vi "参数设置页.vi"() -> ()   [LabVIEW 2016, in "斯坦道总氮.lvlib"]
uses:
  <vilib>/Plasmionique/MB Master/MB_Master/MB_Master.lvclass
panel:
  in  "通讯连接":bool
  out "MB table":enum32{"Serial", "TCP"}(tab)
  in  "请选择串口:":refnum<visa-resource-name>
  in  "IP":string="127.0.0.1"
  in  "PORT":string="1001"
  in  "通信方式选择":enum16{"串口", "TCP"}(ring)
  in  "盐度自动补偿：":bool
  out "盐度补偿值":dbl caption="盐度补偿值："
  in  "刷新":bool
  in  "测量模式":enum16{"水样测量", "零点核查", "跨度核查", "标样核查", "加标回收"}(ring)
  in  "参数下拉列表":u16(ring)
  in  "量程下拉列表":enum16{"低量程", "高量程"}(ring)
  in  "流程路径":path=path "data/流程.xml"
  in  "标样核查量程模式":enum16{"高量程", "低量程", "自动"}(ring) caption="标样核查量程模式："
  in  "加标回收量程模式":enum16{"高量程", "低量程", "自动"}(ring) caption="加标回收量程模式："
  in  "跨度核查量程模式":enum16{"高量程", "低量程", "自动"}(ring) caption="跨度核查量程模式："
  in  "零点核查量程模式":enum16{"高量程", "低量程", "自动"}(ring) caption="零点核查量程模式："
  in  "水样测试量程模式":enum16{"高量程", "低量程", "自动"}(ring) caption="水样测试量程模式："
  out "稀释度":dbl caption="稀释度："
  out "阈值（高->低）":dbl caption="阈值（高->低）："
  out "阈值（低->高）":dbl caption="阈值（低->高）："
  out "量程下限":dbl caption="量程下限："
  out "量程上限":dbl caption="量程上限："
  out "检出限":dbl caption="检出限："
  out "曲线截距":dbl caption="曲线截距：" format="%#.6f"
  out "曲线斜率":dbl caption="曲线斜率：" format="%#.6f"
  out "二次多项式系数":dbl caption="二次多项式系数：" format="%#.6f"
  out "消解时长":dbl caption="消解时长："
  out "消解温度":dbl caption="消解温度："
  out "测量精度":u16 caption="测量精度："
  in  "标样核查标液浓度":dbl caption="标样核查标液浓度："
  in  "跨度核查标液浓度":dbl caption="跨度核查标液浓度："
  in  "零点核查标液浓度":dbl caption="零点核查标液浓度："
  in  "跨度值":dbl caption="跨度值："
  # "ppt"
  # "mg/L"
  # "mg/L"
  # "mg/L"
  # "mg/L"
  # "mg/L"
  # "min"
  # "℃"
  # "mg/L"
  # "mg/L"
  # "mg/L"
  # "mg/L"
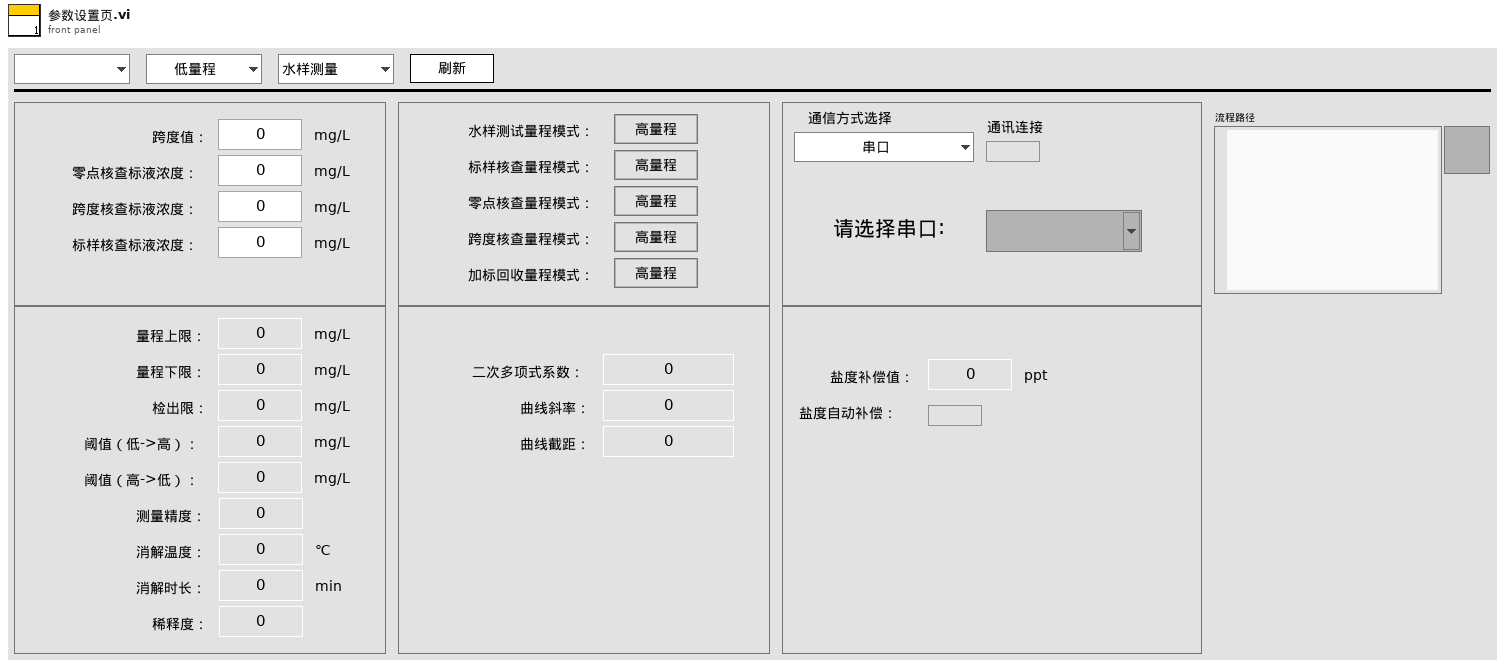
[diagram p1: front panel]
types:
  T1 = typedef "LVStringsAndValuesArrayTypeDef_U16.ctl" = cluster{"String":string, "Value":u16}[]
  T2 = enum8{"Enabled", "Disabled", "Disabled and Grayed Out"}
  T3 = cluster{"泵类型":u8, "进样速度":u32, "出样速度":u32, "泵阀量":u8, "光谱仪类型":u8, "光谱采样次数":u8, "氙灯次数":u8, "B":u16, "C":u16, "D":u16, "E":u16, "B_COD":u16, "C_COD":u16, "D_COD":u16, "E_COD":u16, "G":u16, "M":u16, "N":u16, "氨氮注射泵控温下限":sgl, "氨氮注射泵控温上限":sgl, "总氮注射泵控温下限":sgl, "总氮注射泵控温上限":sgl, "消解温度下限":sgl, "消解温度上限":sgl, "加热10s限值":sgl, "高温高压阀开阀温度":sgl, "总氮x公式0":u8, "总氮x公式1":sgl, "总氮x公式2":sgl, "总磷浊度稀释系数":sgl, "总磷浊度补偿权重1":sgl, "总磷浊度补偿权重2":sgl, "盐度系数":sgl, "氨氮补偿系数1":sgl, "氨氮补偿系数2":sgl}
  T4 = cluster{"测量精度":u16, "检出限":dbl, "上限":dbl, "下限":dbl, "阈值（低->高）":dbl, "阈值（高->低）":dbl, "稀释度":dbl}
  T5 = cluster{"水样测试量程模式":enum16{"高量程", "低量程", "自动"}, "零点核查量程模式":enum16{"高量程", "低量程", "自动"}, "跨度核查量程模式":enum16{"高量程", "低量程", "自动"}, "加标回收量程模式":enum16{"高量程", "低量程", "自动"}, "标样核查量程模式":enum16{"高量程", "低量程", "自动"}}
  T6 = cluster{"总磷跨度值":dbl, "总磷零点标准液浓度":dbl, "总磷跨度标准液浓度":dbl, "总磷标准液标准浓度":dbl, "总氮跨度值":dbl, "总氮零点标准液浓度":dbl, "总氮跨度标准液浓度":dbl, "总氮标准液标准浓度":dbl, "COD跨度值":dbl, "COD零点标准液浓度":dbl, "COD跨度标准液浓度":dbl, "COD标准液标准浓度":dbl, "氨氮跨度值":dbl, "氨氮零点标准液浓度":dbl, "氨氮跨度标准液浓度":dbl, "氨氮标准液标准浓度":dbl, "磷酸盐跨度值":dbl, "磷酸盐零点标准液浓度":dbl, "磷酸盐跨度标准液浓度":dbl, "磷酸盐标准液标准浓度":dbl, "硝氮跨度值":dbl, "硝氮零点标准液浓度":dbl, "硝氮跨度标准液浓度":dbl, "硝氮标准液标准浓度":dbl, "亚硝氮跨度值":dbl, "亚硝氮零点标准液浓度":dbl, "亚硝氮跨度标准液浓度":dbl, "亚硝氮标准液标准浓度":dbl, "硫化物跨度值":dbl, "硫化物零点标准液浓度":dbl, "硫化物跨度标准液浓度":dbl, "硫化物标准液标准浓度":dbl, "硅酸盐跨度值":dbl, "硅酸盐零点标准液浓度":dbl, "硅酸盐跨度标准液浓度":dbl, "硅酸盐标准液标准浓度":dbl}
  T7 = cluster{"水样测试量程模式":u16, "零点核查量程模式":u16, "跨度核查量程模式":u16, "加标回收量程模式":u16, "标样核查量程模式":u16}
  T8 = cluster{"水样测试量程模式":enum16{"H", "L", "AUTO"}, "空白核查量程模式":enum16{"H", "L", "AUTO"}, "跨度核查量程模式":enum16{"H", "L", "AUTO"}, "加标回收量程模式":enum16{"H", "L", "AUTO"}, "标样核查量程模式":enum16{"H", "L", "AUTO"}}
  T9 = cluster{"水样测试量程模式":u16, "空白核查量程模式":u16, "跨度核查量程模式":u16, "加标回收量程模式":u16, "标样核查量程模式":u16}
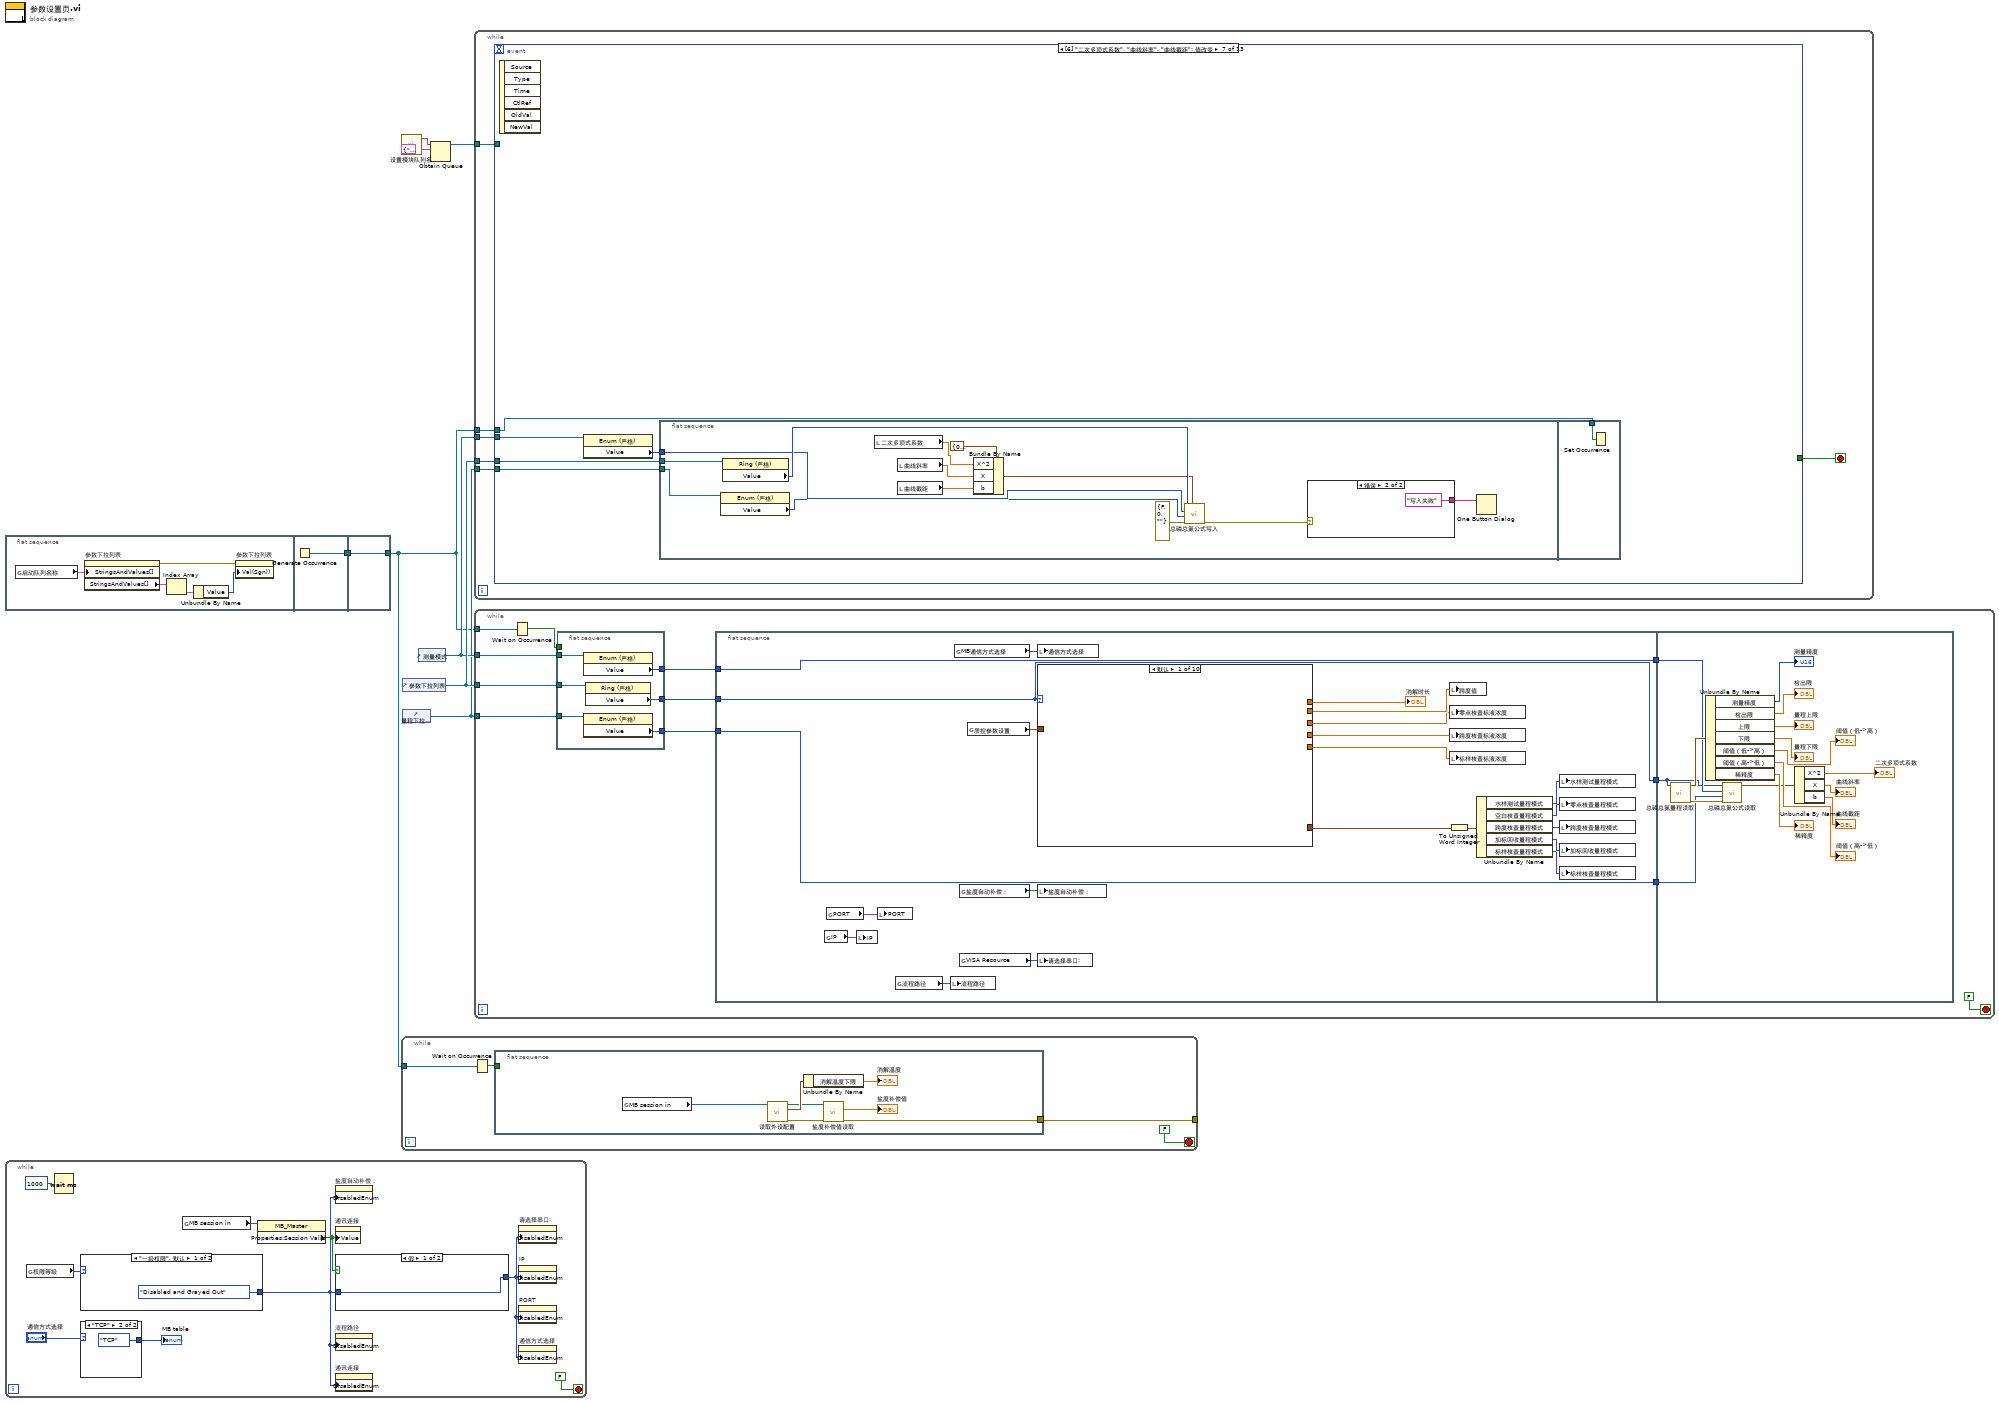
[diagram p0: block diagram]
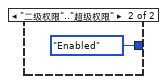
[diagram p2: hidden frame]
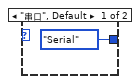
[diagram p3: hidden frame]
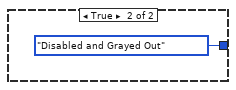
[diagram p4: hidden frame]
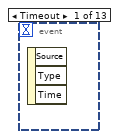
[diagram p5: hidden frame]
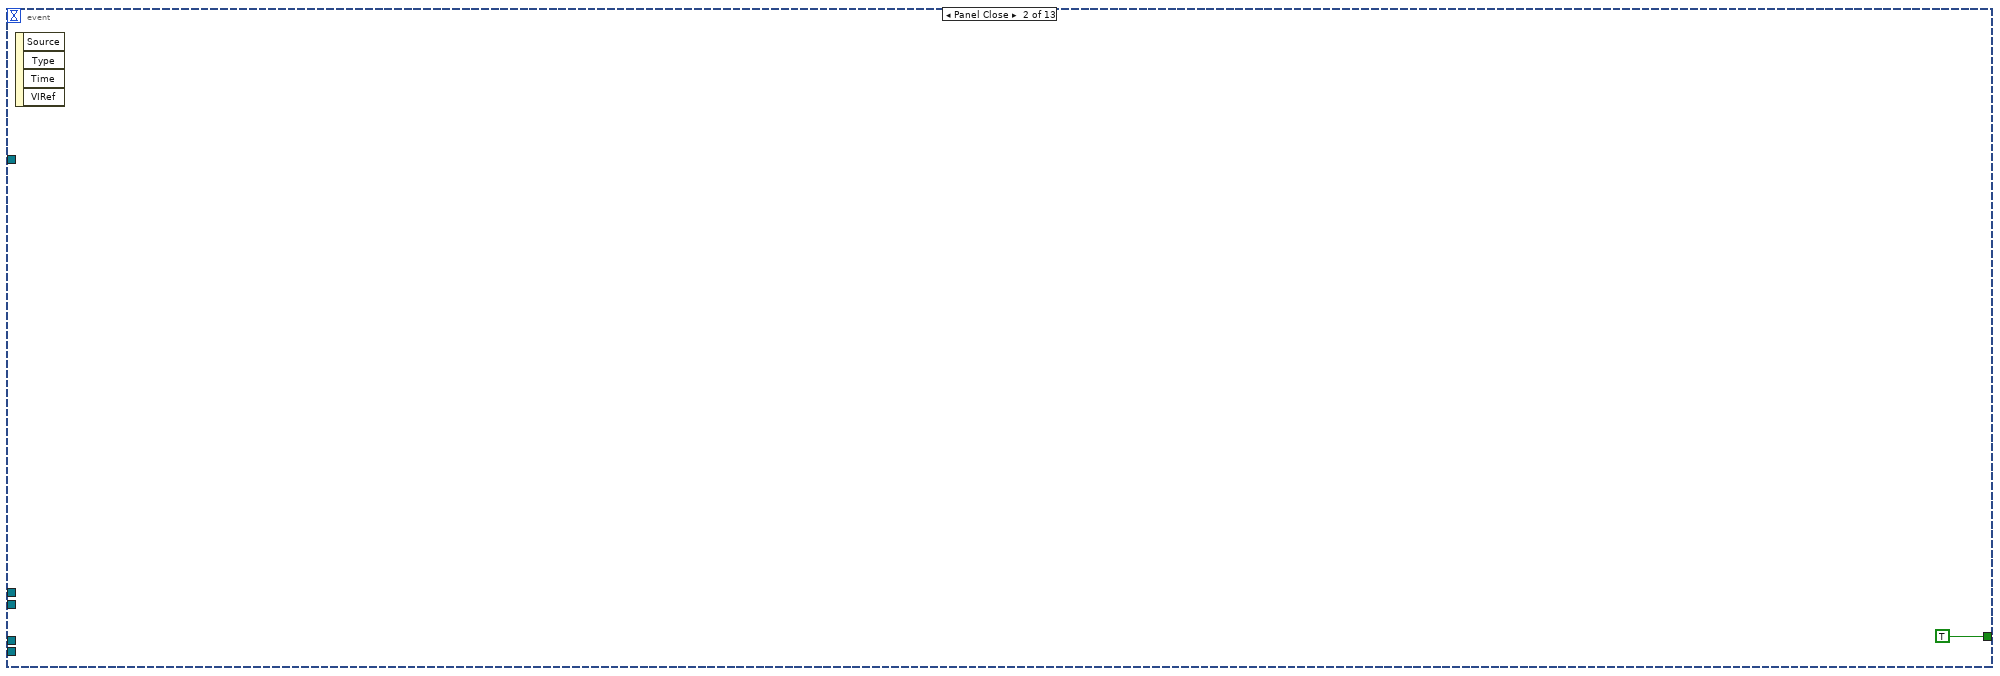
[diagram p6: hidden frame]
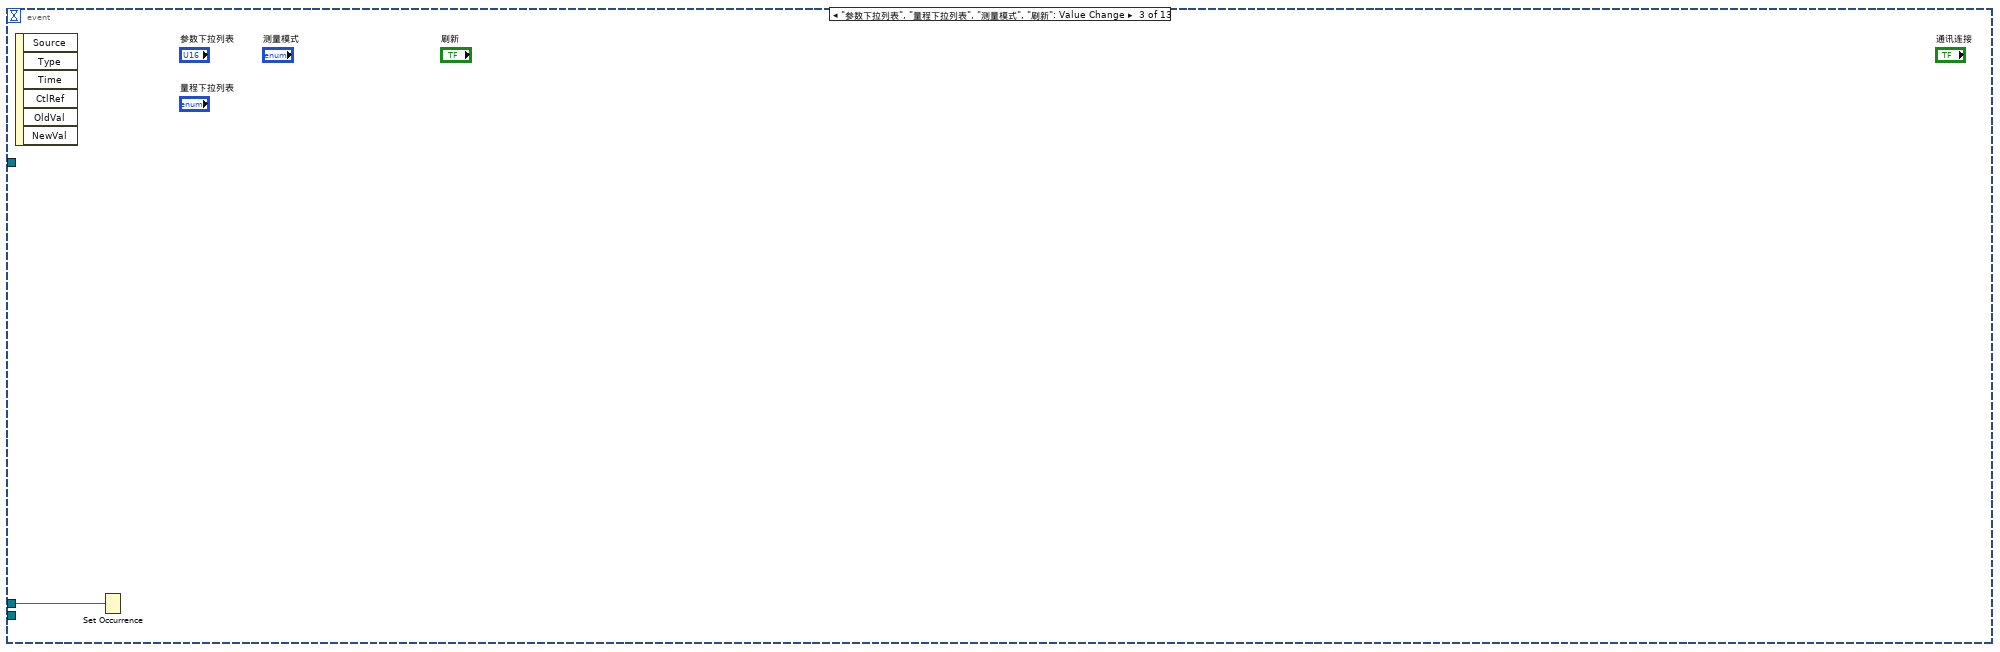
[diagram p7: hidden frame]
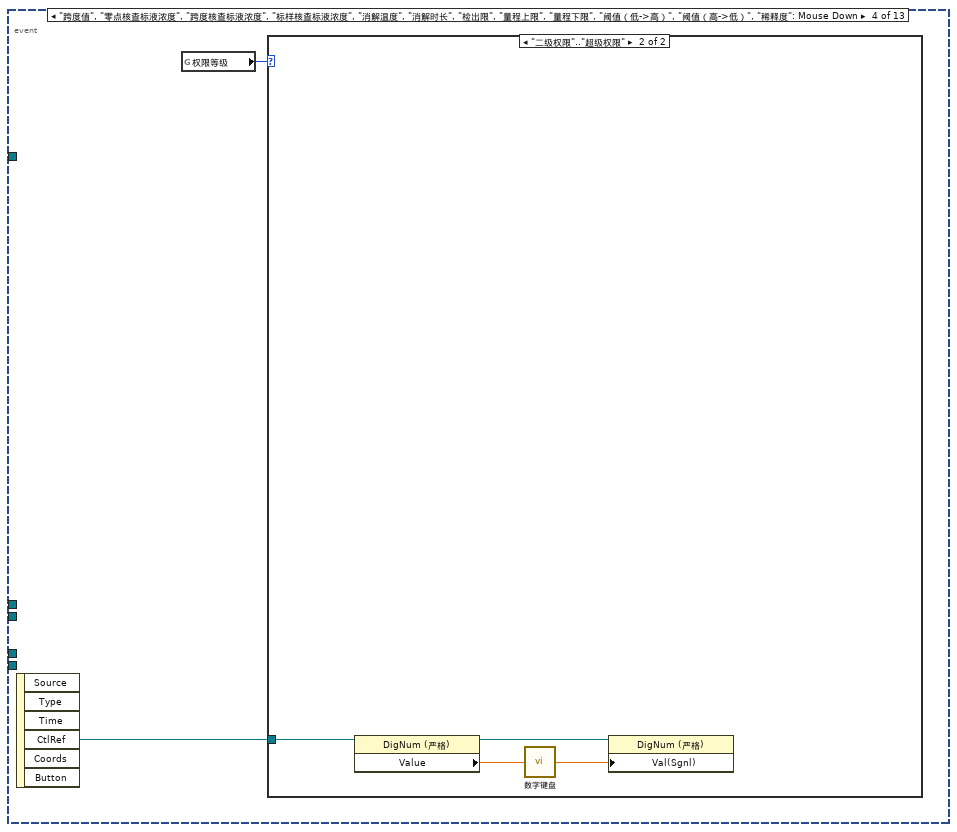
[diagram p8: hidden frame]
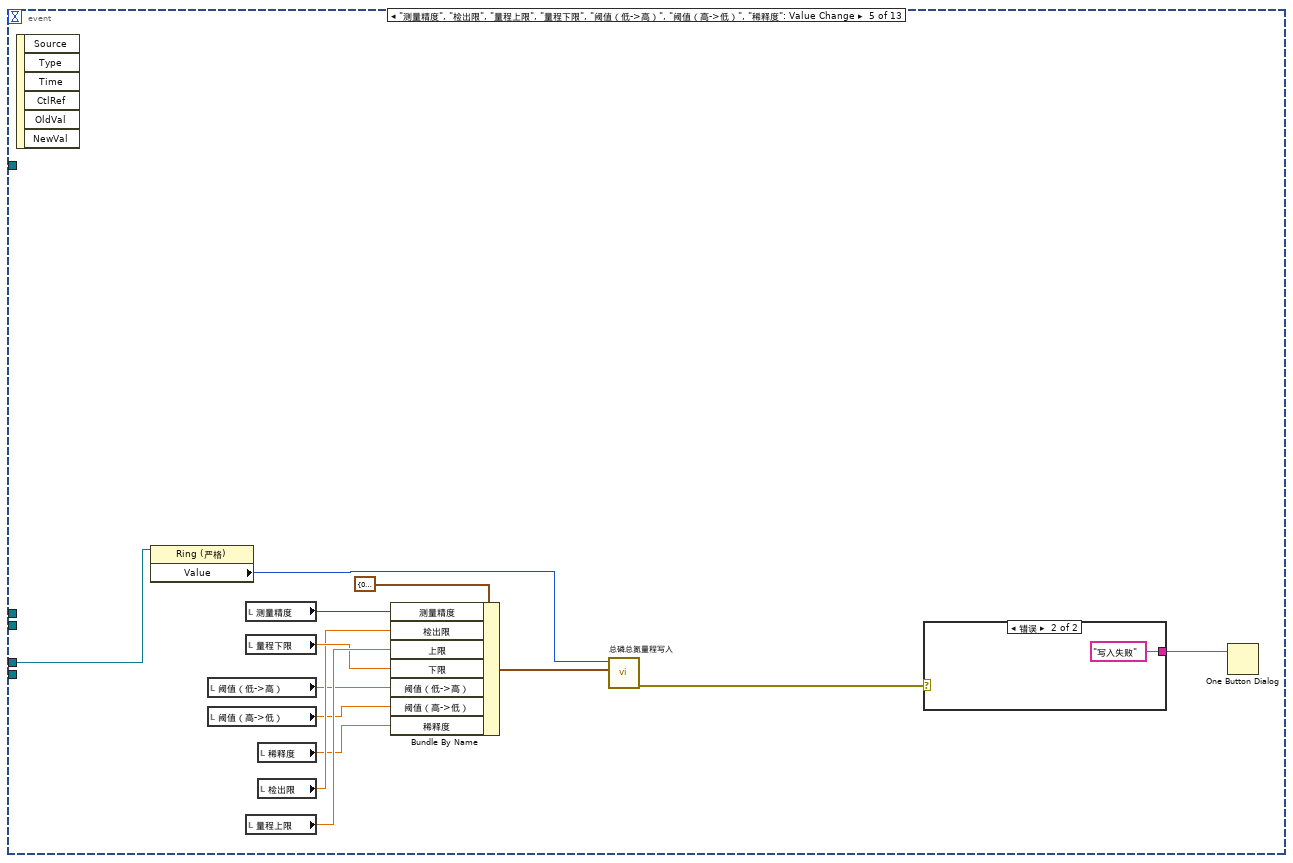
[diagram p10: hidden frame]
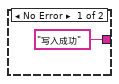
[diagram p11: hidden frame]
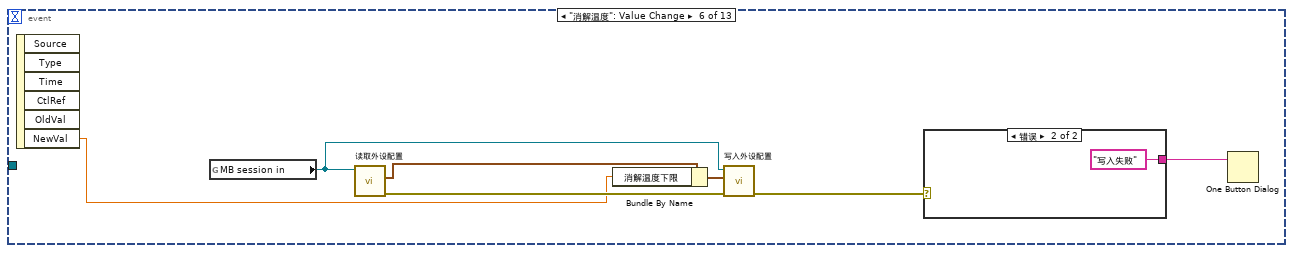
[diagram p12: hidden frame]
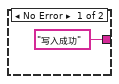
[diagram p13: hidden frame]
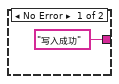
[diagram p14: hidden frame]
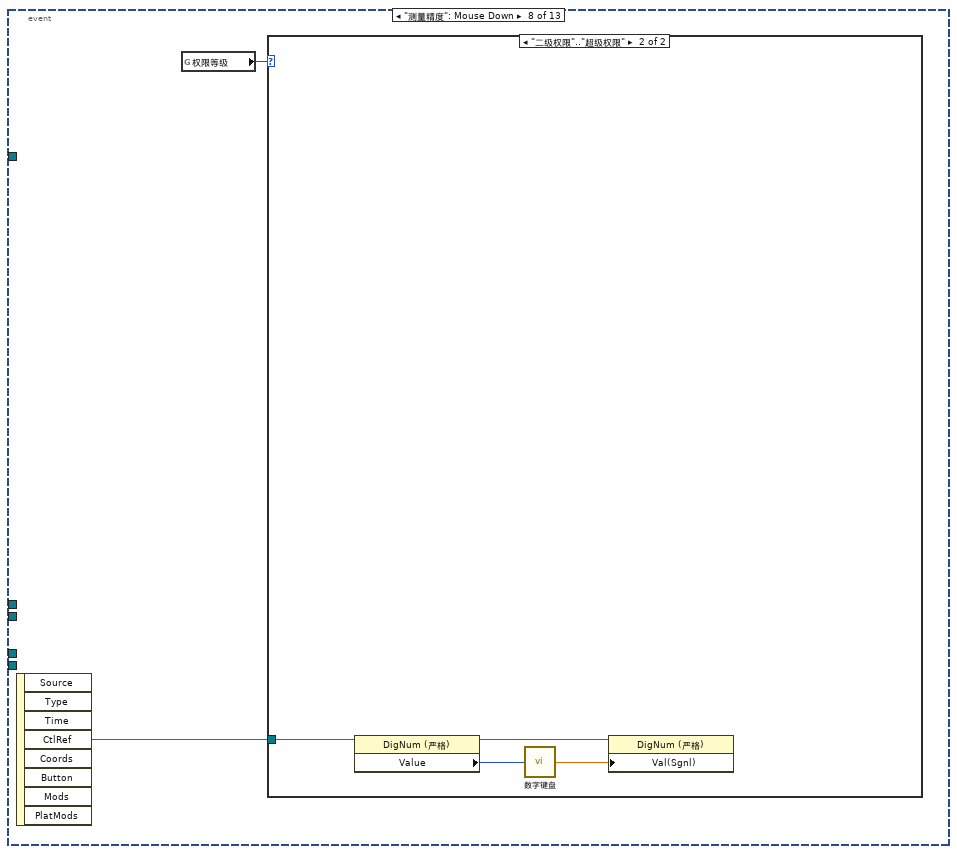
[diagram p15: hidden frame]
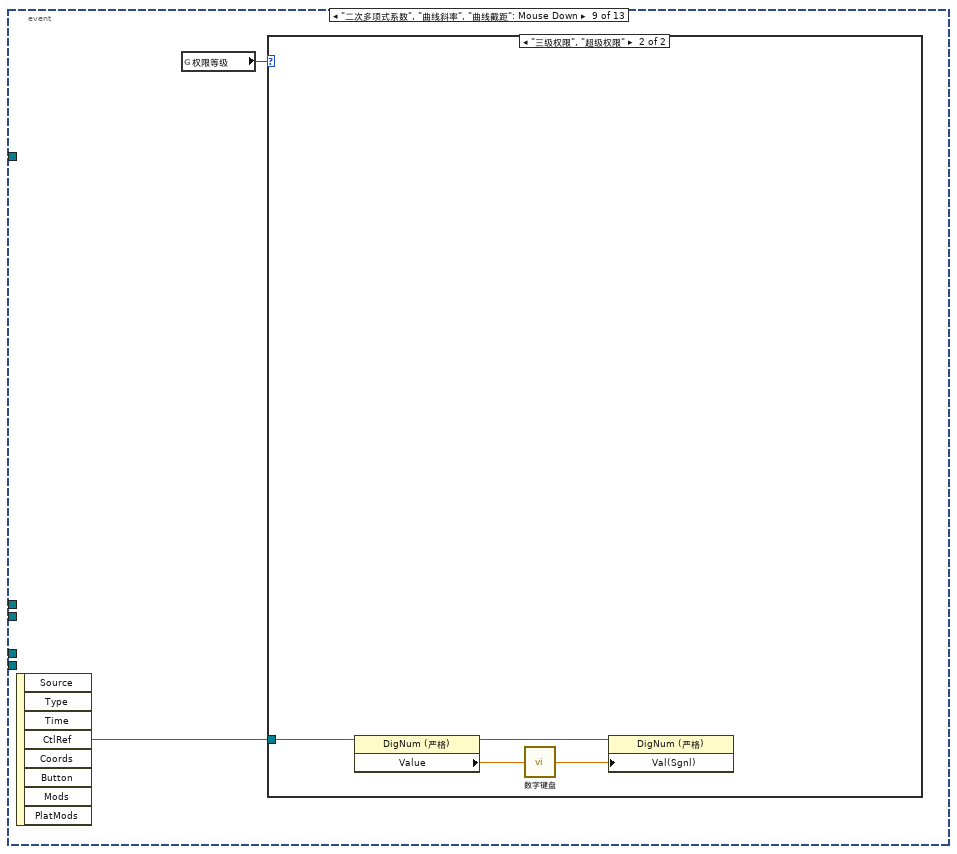
[diagram p17: hidden frame]
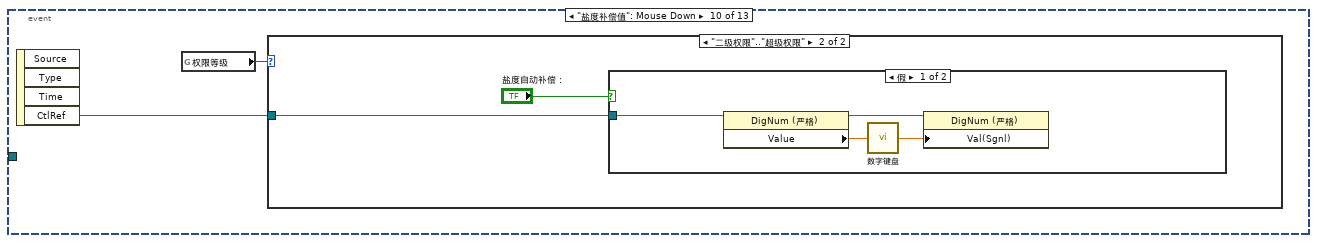
[diagram p19: hidden frame]
diagram:
  n1 = flat-sequence {
    tunnel: [w14] -> w7
    tunnel: [w15] -> w1
    tunnel: w7 -> [w15]
    frame #0 {
      n2 = global read "总磷总氮断电保存全局变量.vi" "启动队列名称"() -> (w9:cluster{"String":string, "Value":u16}[])
      n3 = property on="参数下拉列表" class="Ring (严格)"("StringsAndValues[]"=w9) -> (error out=w12:errorcluster, "StringsAndValues[]"=w10:T1)  [unwired: 2 in, 1 out]
      n4 = Index Array(array=w10) -> (element=w11:cluster{"String":string, "Value":u16})  [unwired: 1 in]
      n5 = Unbundle By Name(w11) -> ("Value"=w13:u16)
      n6 = property on="参数下拉列表" class="Ring (严格)"(error in=w12, "Val(Sgnl)"=w13) -> ()  [unwired: 1 in, 2 out]
    }
    frame #1 {
      n7 = Generate Occurrence() -> (w14:refnum<k4>)
    }
    frame #2 {
    }
  }
  n8 = while {
    stop <- FALSE stop-if-true
    n9 = global read "VAR总磷总氮全局变量.vi" "权限等级"() -> (w16:enum16{"一级权限", "二级权限", "三级权限", "超级权限"})
    n10 = Wait (ms)(milliseconds to wait=u32 1000 ("等待时间（毫秒）")) -> ()  [unwired: 1 out]
    n11 = case shown="\"一级权限\", 默认" w16 {
      tunnel: [T2."Disabled and Grayed Out" ("禁用") T2."Enabled" ("禁用")] -> w17
      frame "一级权限", Default {
      }
      frame "二级权限".."超级权限" {
      }
    }
    n12 = case shown="\"TCP\"" "通信方式选择" {
      tunnel: [enum32{"Serial", "TCP"}."Serial" ("MB table") enum32{"Serial", "TCP"}."TCP" ("MB table")] -> w19
      frame "串口", Default {
      }
      frame "TCP" {
      }
    }
    "MB table" <- w19
    n13 = global read "VAR总磷总氮全局变量.vi" "MB session in"() -> (w23:refnum<class "MB_Master.lvclass">)
    n14 = property class="MB_Master"(reference=w23) -> ("Properties:Session Valid"=w21:bool)  [unwired: 1 in, 2 out]
    n15 = property on="盐度自动补偿：" class="Bool (严格)"("DisabledEnum"=w17) -> ()  [unwired: 2 in, 2 out]
    n16 = property on="通讯连接" class="Bool (严格)"("Value"=w21) -> ()  [unwired: 2 in, 2 out]
    n17 = case shown="假" w21 {
      tunnel: [w29 T2."Disabled and Grayed Out" ("禁用")] -> w20
      tunnel: w17 -> [w29 _]
      frame False {
      }
      frame True {
      }
    }
    n18 = property on="流程路径" class="Path"("DisabledEnum"=w17) -> ()  [unwired: 2 in, 2 out]
    n19 = property on="通讯连接" class="Bool (严格)"("DisabledEnum"=w17) -> ()  [unwired: 2 in, 2 out]
    n20 = property on="请选择串口:" class="VISAName"("DisabledEnum"=w20) -> ()  [unwired: 2 in, 2 out]
    n21 = property on="IP" class="Str"("DisabledEnum"=w20) -> ()  [unwired: 2 in, 2 out]
    n22 = property on="PORT" class="Str"("DisabledEnum"=w20) -> ()  [unwired: 2 in, 2 out]
    n23 = property on="通信方式选择" class="Enum (严格)"("DisabledEnum"=w20) -> ()  [unwired: 2 in, 2 out]
  }
  n24 = call "设置模块队列名.vi"() -> ("Msg"=w5:string)  [unwired: 5 in]
  n25 = while {
    tunnel: [w33] -> _
    tunnel: w1 -> [w32]
    stop <- FALSE stop-if-true
    n26 = Wait on Occurrence(2:w32) -> (0:w31:bool)  [unwired: 2 in]
    n27 = flat-sequence {
      tunnel: [w35] -> w33
      tunnel: w31 -> [_]
      frame #0 {
        n28 = global read "VAR总磷总氮全局变量.vi" "MB session in"() -> (w39:refnum<class "MB_Master.lvclass">)
        n29 = call "读取外设配置.vi"("MB session in"=w39) -> ("error out"=w40:errorcluster, "外设配置"=w37:T3, "MB session out"=w36:refnum<class "MB_Master.lvclass">)  [unwired: 8 in]
        n30 = Unbundle By Name(w37) -> ("消解温度下限"=→"消解温度":sgl)
        n31 = call "盐度补偿值读取.vi"("Error in"=w40, "MB session in"=w36) -> ("error out"=w35:errorcluster, "盐度补偿值"=→"盐度补偿值":sgl)  [unwired: 7 in, 1 out]
      }
    }
  }
  n32 = control-ref of="参数下拉列表"() -> (w8:refnum<vi>)
  n33 = control-ref of="量程下拉列表"() -> (w2:refnum<vi>)
  n34 = control-ref of="测量模式"() -> (w3:refnum<vi>)
  n35 = Obtain Queue(name (unnamed)=w5, element data type=cluster{"命令":string, "data":variant} {"命令"="", "data"=variant}) -> (queue out=w4:refnum<queue>)  [unwired: 3 in, 2 out]
  n36 = while {
    tunnel: w1 -> [w46]
    tunnel: w8 -> [w45]
    tunnel: w4 -> [w44]
    tunnel: w3 -> [w43]
    tunnel: w2 -> [w42]
    stop <- w47 stop-if-true
    n37 = event shown="[6] \"二次多项式系数\", \"曲线斜率\", \"曲线截距\": 值改变" {
      selector: _ -> [_ _ _ _ _ _ _ _ _ _ _ _ _]
      dyn-events: _ -> [_ _ _ _ _ _ _ _ _ _ _ _ _]
      timeout: _ -> [_ _ _ _ _ _ _ _ _ _ _ _ _]
      tunnel: [_ TRUE _ _ _ _ _ _ _ _ _ _ _] -> w47
      tunnel: w46 -> [_ _ w49 _ _ _ w80 _ _ _ _ w123 _]
      tunnel: w45 -> [_ _ _ _ w68 _ w84 _ _ _ _ w125 _]
      tunnel: w44 -> [_ _ _ _ _ _ _ _ _ _ _ _ w215]
      tunnel: w43 -> [_ _ _ _ _ _ w83 _ _ _ _ _ _]
      tunnel: w42 -> [_ _ _ _ _ _ w81 _ _ _ _ _ _]
      event Timeout {
        n38 = event-data() -> ()  [unwired: 1 in, 3 out]
      }
      event Panel Close {
        n39 = event-data() -> ()  [unwired: 1 in, 4 out]
      }
      event "参数下拉列表", "量程下拉列表", "测量模式", "刷新": Value Change {
        n40 = event-data() -> ()  [unwired: 1 in, 6 out]
        n41 = Set Occurrence(w49) -> ()
      }
      event "跨度值", "零点核查标液浓度", "跨度核查标液浓度", "标样核查标液浓度", "消解温度", "消解时长", "检出限", "量程上限", "量程下限", "阈值（低->高）", "阈值（高->低）", "稀释度": Mouse Down {
        n42 = event-data() -> ("CtlRef"=w51:refnum<vi>)  [unwired: 1 in, 5 out]
        n43 = global read "VAR总磷总氮全局变量.vi" "权限等级"() -> (w50:enum16{"一级权限", "二级权限", "三级权限", "超级权限"})
        n44 = case shown="\"二级权限\"..\"超级权限\"" w50 {
          tunnel: w51 -> [_ w55]
          frame "一级权限", Default {
          }
          frame "二级权限".."超级权限" {
            n45 = property class="DigNum (严格)"(reference=w55) -> (reference out=w53:refnum<vi>, "Value"=w54:dbl)  [unwired: 1 in, 1 out]
            n46 = call "数字键盘.vi"("OldNumber"=w54) -> ("NewNumber"=w52:dbl)
            n47 = property class="DigNum (严格)"(reference=w53, "Val(Sgnl)"=w52) -> ()  [unwired: 1 in, 2 out]
          }
        }
      }
      event "测量精度", "检出限", "量程上限", "量程下限", "阈值（低->高）", "阈值（高->低）", "稀释度": Value Change {
        n48 = event-data() -> ()  [unwired: 1 in, 6 out]
        n49 = property class="Ring (严格)"(reference=w68) -> ("Value"=w67:u16)  [unwired: 1 in, 2 out]
        n50 = local read "阈值（低->高）"() -> (w61:dbl)
        n51 = local read "阈值（高->低）"() -> (w60:dbl)
        n52 = local read "测量精度"() -> (w58:u16)
        n53 = local read "量程下限"() -> (w63:dbl)
        n54 = local read "量程上限"() -> (w64:dbl)
        n55 = local read "稀释度"() -> (w59:dbl)
        n56 = local read "检出限"() -> (w62:dbl)
        n57 = Bundle By Name(cluster=T4 {"测量精度"=0, "检出限"=0.0, "上限"=0.0, "下限"=0.0, "阈值（低->高）"=0.0, "阈值（高->低）"=0.0, "稀释度"=0.0} ("量程参数写入"), "测量精度"=w58, "检出限"=w62, "上限"=w64, "下限"=w63, "阈值（低->高）"=w61, "阈值（高->低）"=w60, "稀释度"=w59) -> (w65:T4)
        n58 = call "总磷总氮量程写入.vi"("量程参数写入"=w65, "测量参数"=w67) -> ("error out"=w56:errorcluster)  [unwired: 8 in]
        n59 = case shown="错误" w56 {
          tunnel: ["写入成功" "写入失败"] -> w57
          frame No Error {
          }
          frame Error {
          }
        }
        n60 = One Button Dialog(message=w57) -> ()  [unwired: 1 in, 1 out]
      }
      event "消解温度": Value Change {
        n61 = event-data() -> ("NewVal"=w73:dbl)  [unwired: 1 in, 5 out]
        n62 = global read "VAR总磷总氮全局变量.vi" "MB session in"() -> (w74:refnum<class "MB_Master.lvclass">)
        n63 = call "读取外设配置.vi"("MB session in"=w74) -> ("error out"=w77:errorcluster, "外设配置"=w76:T3)  [unwired: 8 in, 1 out]
        n64 = Bundle By Name(cluster=w76, "消解温度下限"=w73) -> (w75:T3)
        n65 = call "写入外设配置.vi"("error in (no error)"=w77, "外设配置"=w75, "MB session in"=w74) -> ("error out"=w72:errorcluster)  [unwired: 7 in, 1 out]
        n66 = case shown="错误" w72 {
          tunnel: ["写入成功" "写入失败"] -> w71
          frame No Error {
          }
          frame Error {
          }
        }
        n67 = One Button Dialog(message=w71) -> ()  [unwired: 1 in, 1 out]
      }
      event "二次多项式系数", "曲线斜率", "曲线截距": Value Change {
        n68 = event-data() -> ()  [unwired: 1 in, 6 out]
        n69 = property class="Enum (严格)"(reference=w83) -> ("Value"=w82:enum16{"水样测量", "零点核查", "跨度核查", "标样核查", "加标回收"})  [unwired: 1 in, 2 out]
        n70 = flat-sequence {
          tunnel: w84 -> [w97]
          tunnel: w82 -> [w95]
          tunnel: w81 -> [w94]
          tunnel: w80 -> [w100]
          frame #0 {
            n71 = property class="Enum (严格)"(reference=w94) -> ("Value"=w93:enum16{"低量程", "高量程"})  [unwired: 1 in, 2 out]
            n72 = property class="Ring (严格)"(reference=w97) -> ("Value"=w96:u16)  [unwired: 1 in, 2 out]
            n73 = local read "二次多项式系数"() -> (w90:dbl)
            n74 = local read "曲线斜率"() -> (w89:dbl)
            n75 = local read "曲线截距"() -> (w88:dbl)
            n76 = Bundle By Name(cluster=cluster{"X^2":dbl, "X":dbl, "b":dbl} {"X^2"=0.0, "X"=0.0, "b"=0.0} ("公式"), "X^2"=w90, "X"=w89, "b"=w88) -> (w91:cluster{"X^2":dbl, "X":dbl, "b":dbl})
            n77 = call "总磷总氮公式写入.vi"("公式"=w91, "error in (no error)"=errorcluster {"status"=FALSE, "code"=0, "source"=""} ("error out"), "量程"=w93, "测量模式"=w95, "测量参数"=w96) -> ("error out"=w86:errorcluster)  [unwired: 6 in]
            n78 = case shown="错误" w86 {
              tunnel: ["写入成功" "写入失败"] -> w87
              frame No Error {
              }
              frame Error {
              }
            }
            n79 = One Button Dialog(message=w87) -> ()  [unwired: 1 in, 1 out]
          }
          frame #1 {
            n80 = Set Occurrence(w100) -> ()
          }
        }
      }
      event "测量精度": Mouse Down {
        n81 = event-data() -> ("CtlRef"=w102:refnum<vi>)  [unwired: 1 in, 7 out]
        n82 = global read "VAR总磷总氮全局变量.vi" "权限等级"() -> (w101:enum16{"一级权限", "二级权限", "三级权限", "超级权限"})
        n83 = case shown="\"二级权限\"..\"超级权限\"" w101 {
          tunnel: w102 -> [_ w106]
          frame "一级权限", Default {
          }
          frame "二级权限".."超级权限" {
            n84 = property class="DigNum (严格)"(reference=w106) -> (reference out=w104:refnum<vi>, "Value"=w105:u16)  [unwired: 1 in, 1 out]
            n85 = call "数字键盘.vi"("OldNumber"=w105) -> ("NewNumber"=w103:dbl)
            n86 = property class="DigNum (严格)"(reference=w104, "Val(Sgnl)"=w103) -> ()  [unwired: 1 in, 2 out]
          }
        }
      }
      event "二次多项式系数", "曲线斜率", "曲线截距": Mouse Down {
        n87 = event-data() -> ("CtlRef"=w108:refnum<vi>)  [unwired: 1 in, 7 out]
        n88 = global read "VAR总磷总氮全局变量.vi" "权限等级"() -> (w107:enum16{"一级权限", "二级权限", "三级权限", "超级权限"})
        n89 = case shown="\"三级权限\", \"超级权限\"" w107 {
          tunnel: w108 -> [_ w112]
          frame "一级权限", Default {
          }
          frame "三级权限", "超级权限" {
            n90 = property class="DigNum (严格)"(reference=w112) -> (reference out=w110:refnum<vi>, "Value"=w111:dbl)  [unwired: 1 in, 1 out]
            n91 = call "数字键盘.vi"("OldNumber"=w111) -> ("NewNumber"=w109:dbl)
            n92 = property class="DigNum (严格)"(reference=w110, "Val(Sgnl)"=w109) -> ()  [unwired: 1 in, 2 out]
          }
        }
      }
      event "盐度补偿值": Mouse Down {
        n93 = event-data() -> ("CtlRef"=w114:refnum<vi>)  [unwired: 1 in, 3 out]
        n94 = global read "VAR总磷总氮全局变量.vi" "权限等级"() -> (w113:enum16{"一级权限", "二级权限", "三级权限", "超级权限"})
        n95 = case shown="\"二级权限\"..\"超级权限\"" w113 {
          tunnel: w114 -> [_ w116]
          frame "一级权限", Default {
          }
          frame "二级权限".."超级权限" {
            n96 = case shown="假" "盐度自动补偿：" {
              tunnel: w116 -> [w120 _]
              frame False {
                n97 = property class="DigNum (严格)"(reference=w120) -> (reference out=w118:refnum<vi>, "Value"=w119:dbl)  [unwired: 1 in, 1 out]
                n98 = call "数字键盘.vi"("OldNumber"=w119) -> ("NewNumber"=w117:dbl)
                n99 = property class="DigNum (严格)"(reference=w118, "Val(Sgnl)"=w117) -> ()  [unwired: 1 in, 2 out]
              }
              frame True {
              }
            }
          }
        }
      }
      event "盐度补偿值": Value Change {
        n100 = event-data() -> ("NewVal"=w121:dbl)  [unwired: 1 in, 5 out]
        n101 = global read "VAR总磷总氮全局变量.vi" "MB session in"() -> (w122:refnum<class "MB_Master.lvclass">)
        n102 = call "盐度补偿值写入.vi"("盐度补偿值"=w121, "MB session in"=w122) -> ()  [unwired: 8 in, 2 out]
      }
      event "跨度值", "零点核查标液浓度", "跨度核查标液浓度", "标样核查标液浓度", "消解时长", "水样测试量程模式", "零点核查量程模式", "跨度核查量程模式", "加标回收量程模式", "标样核查量程模式", "流程路径", "盐度自动补偿：", "IP", "PORT", "请选择串口:", "通信方式选择": Value Change {
        n103 = event-data() -> ()  [unwired: 1 in, 6 out]
        n104 = global read "VAR总磷总氮全局变量.vi" "权限等级"() -> (w124:enum16{"一级权限", "二级权限", "三级权限", "超级权限"})
        n105 = case shown="\"二级权限\"..\"超级权限\"" w124 {
          tunnel: w125 -> [_ w127]
          tunnel: w123 -> [w126 _]
          frame "一级权限", Default {
            n106 = Set Occurrence(w126) -> ()
          }
          frame "二级权限".."超级权限" {
            n107 = flat-sequence {
              tunnel: w127 -> [w147]
              frame #0 {
                n108 = property class="Ring (严格)"(reference=w147) -> ("Value"=w146:u16)  [unwired: 1 in, 2 out]
                n109 = global write "总磷总氮断电保存全局变量.vi" "PORT"("PORT") -> ()
                n110 = global write "总磷总氮断电保存全局变量.vi" "IP"("IP") -> ()
                n111 = global write "总磷总氮断电保存全局变量.vi" "流程路径"("流程路径") -> ()
                n112 = local read "盐度自动补偿："() -> (w133:bool)
                n113 = local read "通信方式选择"() -> (w129:enum16{"串口", "TCP"})
                n114 = global write "总磷总氮断电保存全局变量.vi" "VISA Resource"("请选择串口:") -> ()
                n115 = global write "总磷总氮断电保存全局变量.vi" "盐度自动补偿："(w133) -> ()
                n116 = global write "总磷总氮断电保存全局变量.vi" "MB通信方式选择"(w129) -> ()
                n117 = Bundle("水样测试量程模式"="水样测试量程模式", "零点核查量程模式"="零点核查量程模式", "跨度核查量程模式"="跨度核查量程模式", "加标回收量程模式"="加标回收量程模式", "标样核查量程模式"="标样核查量程模式") -> (w135:T5)  [unwired: 1 in]
                n118 = global read "总磷总氮断电保存全局变量.vi" "质控参数设置"() -> (w141:T6)
                n119 = local read "消解时长"() -> (w128:dbl)
                n120 = To Unsigned Word Integer(number=w135) -> (unsigned 16bit integer=w134:T7)
                n121 = case shown="1" w146 {
                  tunnel: "跨度值" -> [_ w154 w162 w169 w176 w183 w190 w197 w204 w211]
                  tunnel: "标样核查标液浓度" -> [_ w151 w159 w166 w173 w180 w187 w194 w201 w208]
                  tunnel: "跨度核查标液浓度" -> [_ w152 w160 w167 w174 w181 w188 w195 w202 w209]
                  tunnel: "零点核查标液浓度" -> [_ w153 w161 w168 w175 w182 w189 w196 w203 w210]
                  tunnel: w141 -> [_ w156 w164 w171 w178 w185 w192 w199 w206 w213]
                  tunnel: w134 -> [_ w150 w158 w165 w172 w179 w186 w193 w200 _]
                  tunnel: w128 -> [_ w149 w157 _ _ _ _ _ _ w207]
                  frame 0, Default {
                  }
                  frame 1 {
                    n122 = global write "总磷总氮断电保存全局变量.vi" "总氮消解时长"(w149) -> ()
                    n123 = global write "总磷总氮断电保存全局变量.vi" "总磷自动测试量程配置"(w150) -> ()
                    n124 = Bundle By Name(cluster=w156, "总磷跨度值"=w154, "总磷零点标准液浓度"=w153, "总磷跨度标准液浓度"=w152, "总磷标准液标准浓度"=w151) -> (w155:T6)
                    n125 = global write "总磷总氮断电保存全局变量.vi" "质控参数设置"(w155) -> ()
                  }
                  frame 2 {
                    n126 = global write "总磷总氮断电保存全局变量.vi" "总氮消解时长"(w157) -> ()
                    n127 = global write "总磷总氮断电保存全局变量.vi" "总氮自动测试量程配置"(w158) -> ()
                    n128 = Bundle By Name(cluster=w164, "总氮跨度值"=w162, "总氮零点标准液浓度"=w161, "总氮跨度标准液浓度"=w160, "总氮标准液标准浓度"=w159) -> (w163:T6)
                    n129 = global write "总磷总氮断电保存全局变量.vi" "质控参数设置"(w163) -> ()
                  }
                  frame 3 {
                    n130 = global write "总磷总氮断电保存全局变量.vi" "氨氮自动测试量程配置"(w165) -> ()
                    n131 = Bundle By Name(cluster=w171, "氨氮跨度值"=w169, "氨氮零点标准液浓度"=w168, "氨氮跨度标准液浓度"=w167, "氨氮标准液标准浓度"=w166) -> (w170:T6)
                    n132 = global write "总磷总氮断电保存全局变量.vi" "质控参数设置"(w170) -> ()
                  }
                  frame 4 {
                    n133 = Bundle By Name(cluster=w178, "磷酸盐跨度值"=w176, "磷酸盐零点标准液浓度"=w175, "磷酸盐跨度标准液浓度"=w174, "磷酸盐标准液标准浓度"=w173) -> (w177:T6)
                    n134 = global write "总磷总氮断电保存全局变量.vi" "磷酸盐自动测试量程配置"(w172) -> ()
                    n135 = global write "总磷总氮断电保存全局变量.vi" "质控参数设置"(w177) -> ()
                  }
                  frame 5 {
                    n136 = global write "总磷总氮断电保存全局变量.vi" "硝氮自动测试量程配置"(w179) -> ()
                    n137 = Bundle By Name(cluster=w185, "硝氮跨度值"=w183, "硝氮零点标准液浓度"=w182, "硝氮跨度标准液浓度"=w181, "硝氮标准液标准浓度"=w180) -> (w184:T6)
                    n138 = global write "总磷总氮断电保存全局变量.vi" "质控参数设置"(w184) -> ()
                  }
                  frame 6 {
                    n139 = Bundle By Name(cluster=w192, "亚硝氮跨度值"=w190, "亚硝氮零点标准液浓度"=w189, "亚硝氮跨度标准液浓度"=w188, "亚硝氮标准液标准浓度"=w187) -> (w191:T6)
                    n140 = global write "总磷总氮断电保存全局变量.vi" "亚硝氮自动测试量程配置"(w186) -> ()
                    n141 = global write "总磷总氮断电保存全局变量.vi" "质控参数设置"(w191) -> ()
                  }
                  frame 7 {
                    n142 = Bundle By Name(cluster=w199, "硅酸盐跨度值"=w197, "硅酸盐零点标准液浓度"=w196, "硅酸盐跨度标准液浓度"=w195, "硅酸盐标准液标准浓度"=w194) -> (w198:T6)
                    n143 = global write "总磷总氮断电保存全局变量.vi" "硅酸盐自动测试量程配置"(w193) -> ()
                    n144 = global write "总磷总氮断电保存全局变量.vi" "质控参数设置"(w198) -> ()
                  }
                  frame 8 {
                    n145 = Bundle By Name(cluster=w206, "硫化物跨度值"=w204, "硫化物零点标准液浓度"=w203, "硫化物跨度标准液浓度"=w202, "硫化物标准液标准浓度"=w201) -> (w205:T6)
                    n146 = global write "总磷总氮断电保存全局变量.vi" "硫化物自动测试量程配置"(w200) -> ()
                    n147 = global write "总磷总氮断电保存全局变量.vi" "质控参数设置"(w205) -> ()
                  }
                  frame 22 {
                    n148 = global write "总磷总氮断电保存全局变量.vi" "CODcr消解时长"(w207) -> ()
                    n149 = Bundle By Name(cluster=w213, "COD跨度值"=w211, "COD零点标准液浓度"=w210, "COD跨度标准液浓度"=w209, "COD标准液标准浓度"=w208) -> (w212:T6)
                    n150 = global write "总磷总氮断电保存全局变量.vi" "质控参数设置"(w212) -> ()
                  }
                }
              }
              frame #1 {
                n151 = call "配置写入.vi"() -> ()  [unwired: 11 in, 1 out]
              }
            }
          }
        }
      }
      event "通讯连接": Value Change {
        n152 = event-data() -> ("NewVal"=w214:bool)  [unwired: 1 in, 5 out]
        n153 = Flush Queue(queue=w215) -> (queue out=w216:refnum<queue>)  [unwired: 1 in, 2 out]
        n154 = case shown="真" w214 {
          tunnel: w216 -> [w217 w219]
          frame False {
            n155 = Enqueue Element(queue=w217, element=cluster{"命令":string, "data":variant} {"命令"="停用模块", "data"=variant} ("元素")) -> ()  [unwired: 2 in, 3 out]
          }
          frame True {
            n156 = Enqueue Element(queue=w219, element=cluster{"命令":string, "data":variant} {"命令"="启用模块", "data"=variant} ("元素")) -> ()  [unwired: 2 in, 3 out]
          }
        }
      }
    }
  }
  n157 = while {
    tunnel: w8 -> [w231]
    tunnel: w2 -> [w230]
    tunnel: w3 -> [w229]
    tunnel: w1 -> [w228]
    stop <- FALSE stop-if-true
    n158 = Wait on Occurrence(2:w228) -> (0:w221:bool)  [unwired: 2 in]
    n159 = flat-sequence {
      tunnel: w231 -> [w238]
      tunnel: w230 -> [w237]
      tunnel: w229 -> [w236]
      tunnel: [w235] -> w224
      tunnel: [w234] -> w223
      tunnel: [w233] -> w222
      tunnel: w221 -> [_]
      frame #0 {
        n160 = property class="Enum (严格)"(reference=w236) -> ("Value"=w233:enum16{"水样测量", "零点核查", "跨度核查", "标样核查", "加标回收"})  [unwired: 1 in, 2 out]
        n161 = property class="Enum (严格)"(reference=w237) -> ("Value"=w234:enum16{"低量程", "高量程"})  [unwired: 1 in, 2 out]
        n162 = property class="Ring (严格)"(reference=w238) -> ("Value"=w235:u16)  [unwired: 1 in, 2 out]
      }
    }
    n163 = flat-sequence {
      tunnel: [w252] -> w227
      tunnel: [w260] -> w226
      tunnel: [w251] -> w225
      tunnel: w224 -> [w252]
      tunnel: w223 -> [w260]
      tunnel: w222 -> [w251]
      tunnel: w227 -> [w318]
      tunnel: w226 -> [w319]
      tunnel: w225 -> [w320]
      frame #0 {
        n164 = global read "总磷总氮断电保存全局变量.vi" "IP"() -> (w248:string)
        n165 = global read "总磷总氮断电保存全局变量.vi" "PORT"() -> (w247:string)
        n166 = local write "IP"(w248) -> ()
        n167 = local write "PORT"(w247) -> ()
        n168 = global read "总磷总氮断电保存全局变量.vi" "流程路径"() -> (w249:path)
        n169 = local write "流程路径"(w249) -> ()
        n170 = global read "总磷总氮断电保存全局变量.vi" "MB通信方式选择"() -> (w246:enum16{"串口", "TCP"})
        n171 = global read "总磷总氮断电保存全局变量.vi" "盐度自动补偿："() -> (w250:bool)
        n172 = global read "总磷总氮断电保存全局变量.vi" "VISA Resource"() -> (w245:refnum<visa-resource-name>)
        n173 = global read "总磷总氮断电保存全局变量.vi" "质控参数设置"() -> (w243:T6)
        n174 = local write "通信方式选择"(w246) -> ()
        n175 = case shown="默认" w252 {
          tunnel: [_ w267 w274 w280 w286 w292 w298 w304 w310 w317] -> w253
          tunnel: [_ w266 w273 _ _ _ _ _ _ w316] -> w244
          tunnel: w243 -> [_ w265 w272 w279 w285 w291 w297 w303 w309 w315]
          tunnel: [_ w264 w271 w278 w284 w290 w296 w302 w308 w314] -> w242
          tunnel: [_ w263 w270 w277 w283 w289 w295 w301 w307 w313] -> w241
          tunnel: [_ w262 w269 w276 w282 w288 w294 w300 w306 w312] -> w240
          tunnel: [_ w261 w268 w275 w281 w287 w293 w299 w305 w311] -> w239
          frame Default {
          }
          frame 1 {
            n176 = Unbundle By Name(w265) -> ("总磷跨度值"=w264:dbl, "总磷零点标准液浓度"=w263:dbl, "总磷跨度标准液浓度"=w262:dbl, "总磷标准液标准浓度"=w261:dbl)
            n177 = global read "总磷总氮断电保存全局变量.vi" "总磷自动测试量程配置"() -> (w267:T8)
            n178 = global read "总磷总氮断电保存全局变量.vi" "总磷消解时长"() -> (w266:dbl)
          }
          frame 2 {
            n179 = Unbundle By Name(w272) -> ("总氮跨度值"=w271:dbl, "总氮零点标准液浓度"=w270:dbl, "总氮跨度标准液浓度"=w269:dbl, "总氮标准液标准浓度"=w268:dbl)
            n180 = global read "总磷总氮断电保存全局变量.vi" "总氮自动测试量程配置"() -> (w274:T8)
            n181 = global read "总磷总氮断电保存全局变量.vi" "总氮消解时长"() -> (w273:dbl)
          }
          frame 3 {
            n182 = Unbundle By Name(w279) -> ("氨氮跨度值"=w278:dbl, "氨氮零点标准液浓度"=w277:dbl, "氨氮跨度标准液浓度"=w276:dbl, "氨氮标准液标准浓度"=w275:dbl)
            n183 = global read "总磷总氮断电保存全局变量.vi" "氨氮自动测试量程配置"() -> (w280:T8)
          }
          frame 4 {
            n184 = Unbundle By Name(w285) -> ("磷酸盐跨度值"=w284:dbl, "磷酸盐零点标准液浓度"=w283:dbl, "磷酸盐跨度标准液浓度"=w282:dbl, "磷酸盐标准液标准浓度"=w281:dbl)
            n185 = global read "总磷总氮断电保存全局变量.vi" "磷酸盐自动测试量程配置"() -> (w286:T8)
          }
          frame 5 {
            n186 = Unbundle By Name(w291) -> ("硝氮跨度值"=w290:dbl, "硝氮零点标准液浓度"=w289:dbl, "硝氮跨度标准液浓度"=w288:dbl, "硝氮标准液标准浓度"=w287:dbl)
            n187 = global read "总磷总氮断电保存全局变量.vi" "硝氮自动测试量程配置"() -> (w292:T8)
          }
          frame 6 {
            n188 = Unbundle By Name(w297) -> ("亚硝氮跨度值"=w296:dbl, "亚硝氮零点标准液浓度"=w295:dbl, "亚硝氮跨度标准液浓度"=w294:dbl, "亚硝氮标准液标准浓度"=w293:dbl)
            n189 = global read "总磷总氮断电保存全局变量.vi" "亚硝氮自动测试量程配置"() -> (w298:T8)
          }
          frame 7 {
            n190 = Unbundle By Name(w303) -> ("硅酸盐跨度值"=w302:dbl, "硅酸盐零点标准液浓度"=w301:dbl, "硅酸盐跨度标准液浓度"=w300:dbl, "硅酸盐标准液标准浓度"=w299:dbl)
            n191 = global read "总磷总氮断电保存全局变量.vi" "硅酸盐自动测试量程配置"() -> (w304:T8)
          }
          frame 8 {
            n192 = Unbundle By Name(w309) -> ("硫化物跨度值"=w308:dbl, "硫化物零点标准液浓度"=w307:dbl, "硫化物跨度标准液浓度"=w306:dbl, "硫化物标准液标准浓度"=w305:dbl)
            n193 = global read "总磷总氮断电保存全局变量.vi" "硫化物自动测试量程配置"() -> (w310:T8)
          }
          frame 22 {
            n194 = Unbundle By Name(w315) -> ("COD跨度值"=w314:dbl, "COD零点标准液浓度"=w313:dbl, "COD跨度标准液浓度"=w312:dbl, "COD标准液标准浓度"=w311:dbl)
            n195 = global read "总磷总氮断电保存全局变量.vi" "COD自动测试量程配置"() -> (w317:T8)
            n196 = global read "总磷总氮断电保存全局变量.vi" "CODcr消解时长"() -> (w316:dbl)
          }
        }
        "消解时长" <- w244
        n197 = local write "盐度自动补偿："(w250) -> ()
        n198 = local write "请选择串口:"(w245) -> ()
        n199 = local write "跨度值"(w242) -> ()
        n200 = local write "零点核查标液浓度"(w241) -> ()
        n201 = local write "跨度核查标液浓度"(w240) -> ()
        n202 = local write "标样核查标液浓度"(w239) -> ()
        n203 = To Unsigned Word Integer(number=w253) -> (unsigned 16bit integer=w254:T9)
        n204 = Unbundle By Name(w254) -> ("水样测试量程模式"=w255:u16, "空白核查量程模式"=w257:u16, "跨度核查量程模式"=w258:u16, "加标回收量程模式"=w259:u16, "标样核查量程模式"=w256:u16)
        n205 = local write "水样测试量程模式"(w255) -> ()
        n206 = local write "零点核查量程模式"(w257) -> ()
        n207 = local write "跨度核查量程模式"(w258) -> ()
        n208 = local write "加标回收量程模式"(w259) -> ()
        n209 = local write "标样核查量程模式"(w256) -> ()
      }
      frame #1 {
        n210 = call "总磷总氮量程读取.vi"("测量参数"=w318) -> ("error out"=w325:errorcluster, "量程参数读取"=w333:T4)  [unwired: 9 in]
        n211 = Unbundle By Name(w333) -> ("测量精度"=→"测量精度":u16, "检出限"=→"检出限":dbl, "上限"=→"量程上限":dbl, "下限"=→"量程下限":dbl, "阈值（低->高）"=→"阈值（低->高）":dbl, "阈值（高->低）"=→"阈值（高->低）":dbl, "稀释度"=→"稀释度":dbl)
        n212 = call "总磷总氮公式读取.vi"("error in (no error)"=w325, "量程"=w319, "测量模式"=w320, "测量参数"=w318) -> ("公式"=w324:cluster{"X^2":dbl, "X":dbl, "b":dbl})  [unwired: 6 in, 1 out]
        n213 = Unbundle By Name(w324) -> ("X^2"=→"二次多项式系数":dbl, "X"=→"曲线斜率":dbl, "b"=→"曲线截距":dbl)
      }
    }
  }
